vi "ActionVIOnCompile.vi"(8 "error in (no error)":errorcluster, 11 "Device Item Ref in":T1 format="%.0x") -> (0 "error out":errorcluster)   [LabVIEW 2020, in "Waveform-Processing-Custom-Device System Explorer.lvlib"]
uses:
  Waveform-Processing-Custom-Device System Explorer.lvlib
  <vilib>/NI VeriStand/Custom Device API/Custom Device Item Ref.ctl
  Shared/Types/FG Action.ctl
  Shared/CompiledSettings.ctl
  <vilib>/NI VeriStand/Custom Device API/Block Data Reference.ctl
  <vilib>/NI VeriStand/Custom Device API/Data Reference.ctl
  <vilib>/NI VeriStand/Custom Device API/Waveform Data Reference.ctl
  Shared/Constants.vi
  <vilib>/NI VeriStand/Custom Device API/Set Item Property (Variant).vi
  <vilib>/NI VeriStand/Custom Device API/Custom Device API.lvlib
  <vilib>/NI/NIVS Inline Async API/_Data Access System Explorer/Data Access System Explorer.lvlib
  Shared/Waveform-Processing-Custom-Device Shared.lvlib
  Shared/Running Average/Running Average.lvlib
  Shared/Single Point/SinglePoint.lvlib
  Shared/Scaled Waveform/Scaled Waveform.lvlib
  Shared/Debug/Debug.lvlib
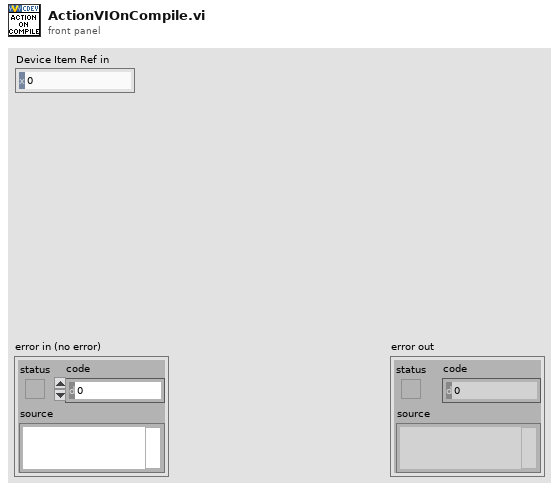
[diagram p1: front panel]
types:
  T1 = typedef "Custom Device API.lvlib/Custom Device Item Ref.ctl" = u64
  T2 = typedef "Waveform-Processing-Custom-Device Shared.lvlib/CompiledSettings.ctl" = cluster{"Name":string, "Buffer Length (samples)":u32, "Enable Array":bool[], "Parameter Block Data Refs":T3[], "Source Wfm Data Refs":T5[], "Result Wfm Data Refs":T5[], "Result Ch Data Refs":T4[], "Task Rate (Hz)":dbl}
  T3 = typedef "Custom Device API.lvlib/Block Data Reference.ctl" = cluster{"Data Reference":T4, "Offset":u64, "Length":u64}
  T4 = typedef "Custom Device API.lvlib/Data Reference.ctl" = i32
  T5 = typedef "Custom Device API.lvlib/Waveform Data Reference.ctl" = i32
  T6 = typedef "Waveform-Processing-Custom-Device Shared.lvlib/FG Action.ctl" = enum8{"GET", "SET"}
  T7 = typedef "Custom Device API.lvlib/Custom Device Item Info.ctl" = cluster{"Name":string, "Is Channel":bool, "GUID":string, "Is Waveform":bool}
  T8 = typedef "Waveform-Processing-Custom-Device Shared.lvlib/Custom Device Settings.ctl" = cluster{"CD Task Dependency":T1, "CD Task Dependency Ref":T1, "CD Task Available Wfms":string[], "CD Task Selected Wfms":string[], "Buffer Length (s)":dbl, "Buffer Length (samples)":u32, "Single-point Enabled":bool, "Running Average Enabled":bool, "Task Rate":dbl, "Scaled Waveform Enabled":bool}
  T9 = cluster{"Name":string, "Type":enum16{"Output/Write", "Input/Read", "Input/ReadWrite"}, "VS Refs":T1[]}[]
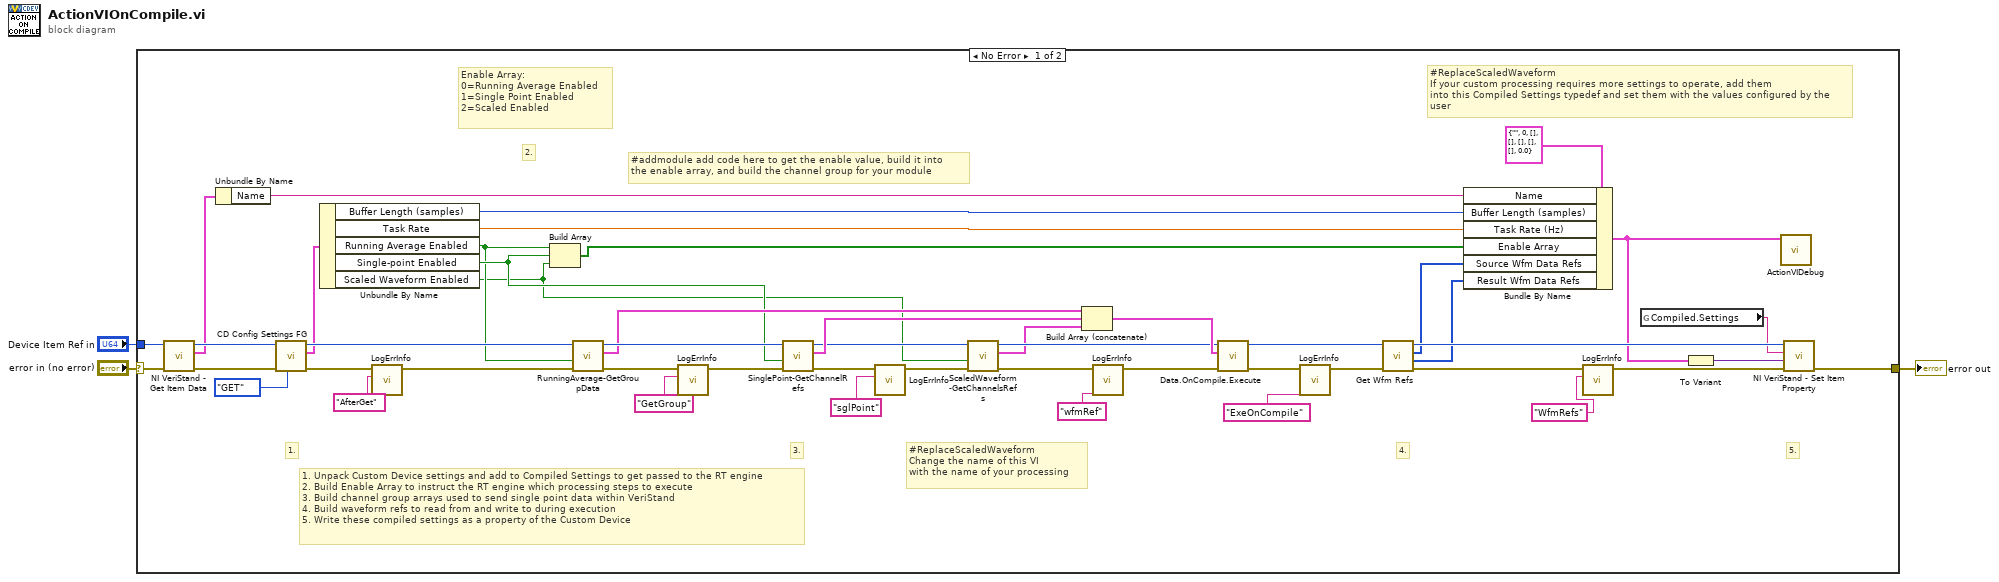
[diagram p0: block diagram]
diagram:
  n1 = case shown="No Error" "error in (no error)" {
    selector: "error in (no error)" -> [w51 w53]
    tunnel: [w52 w53] -> w2
    tunnel: "Device Item Ref in" -> [w50 _]
    frame No Error {
      # "#ReplaceScaledWaveform \nIf your custom processing requires more settings to operate, add them\ninto this Compiled Settings typedef and set them with the values configured by the user"
      # "#ReplaceScaledWaveform \nChange the name of this VI\nwith the name of your processing"
      # "#addmodule add code here to get the enable value, build it into\nthe enable array, and build the channel group for your module"
      # "Enable Array:\n0=Running Average Enabled\n1=Single Point Enabled\n2=Scaled Enabled"
      # "5."
      # "4."
      # "3."
      # "2."
      # "1."
      # "1. Unpack Custom Device settings and add to Compiled Settings to get passed to the RT engine\n2. Build Enable Array to instruct the RT engine which processing steps to execute\n3. Build channel group arrays used to send single point data within VeriStand\n4. Build waveform refs to read from and write to during execution\n5. Write these compiled settings as a property of the Custom Device"
      n2 = call <vilib>:"NI VeriStand - Get Item Data.vi"("error in (no error)"=w51, "Item Ref in"=w50) -> ("error out"=w48:errorcluster, "Item Info"=w47:T7, "Item Ref out"=w49:T1)  [unwired: 6 in, 1 out]
      n3 = Unbundle By Name(w47) -> ("Name"=w38:string)
      n4 = call "CD Config Settings FG.vi"("Action"=FG_Action."GET", "error in (no error)"=w48, "Item Ref"=w49) -> ("error out"=w16:errorcluster, "CD Settings out"=w37:T8, "Item Ref out"=w41:T1)  [unwired: 5 in, 1 out]
      n5 = Unbundle By Name(w37) -> ("Buffer Length (samples)"=w36:u32, "Task Rate"=w27:dbl, "Running Average Enabled"=w29:bool, "Single-point Enabled"=w30:bool, "Scaled Waveform Enabled"=w18:bool)
      n6 = call "LogErrInfo.vi"("location info"="AfterGet", "error in (no error)"=w16) -> ("error out"=w15:errorcluster)  [unwired: 9 in]
      n7 = Build Array(w29, w30, w18) -> (w28:bool[])
      n8 = call "RunningAverage-GetGroupData.vi"("Error in"=w15, "Enabled?"=w29, "Device Ref in"=w41) -> ("Error out"=w45:errorcluster, "Group Data Array"=w35:T9, "Device Ref out"=w40:T1)  [unwired: 6 in]
      n9 = call "LogErrInfo.vi"("location info"="GetGroup", "error in (no error)"=w45) -> ("error out"=w13:errorcluster)  [unwired: 9 in]
      n10 = call "SinglePoint-GetChannelRefs.vi"("Error in"=w13, "Enabled?"=w30, "Device Ref in"=w40) -> ("Error out"=w22:errorcluster, "Group Data Array"=w34:T9, "Device Ref out"=w19:T1)  [unwired: 6 in]
      n11 = call "LogErrInfo.vi"("location info"="sglPoint", "error in (no error)"=w22) -> ("error out"=w11:errorcluster)  [unwired: 9 in]
      n12 = call "ScaledWaveform-GetChannelsRefs.vi"("Error in"=w11, "Enabled?"=w18, "Device Ref in"=w19) -> ("Error out"=w21:errorcluster, "Group Data Array"=w17:T9, "Device Ref out"=w20:T1)  [unwired: 6 in]
      n13 = Build Array (concatenate)(w35, w34, w17) -> (w31:T9)
      n14 = call "LogErrInfo.vi"("location info"="wfmRef", "error in (no error)"=w21) -> ("error out"=w10:errorcluster)  [unwired: 9 in]
      n15 = call <vilib>:"Data.OnCompile.Execute.vi"("error in"=w10, "VS Ref Groups"=w31, "Custom Device Ref"=w20) -> ("error out"=w32:errorcluster, "Custom Device Ref"=w33:T1)  [unwired: 7 in]
      n16 = call "LogErrInfo.vi"("location info"="ExeOnCompile", "error in (no error)"=w32) -> ("error out"=w9:errorcluster)  [unwired: 9 in]
      n17 = call "Get Wfm Refs.vi"("Error in"=w9, "Device Ref in"=w33) -> ("Error out"=w44:errorcluster, "Results Wfm Data Refs"=w25:T5[], "Source Wfm Data Refs"=w26:T5[], "Device Ref out"=w39:T1)  [unwired: 6 in]
      n18 = Bundle By Name(cluster=T2 {"Name"="", "Buffer Length (samples)"=0, "Enable Array"=[], "Parameter Block Data Refs"=[], "Source Wfm Data Refs"=[], "Result Wfm Data Refs"=[], "Result Ch Data Refs"=[], "Task Rate (Hz)"=0.0} ("CompiledSettings"), "Name"=w38, "Buffer Length (samples)"=w36, "Task Rate (Hz)"=w27, "Enable Array"=w28, "Source Wfm Data Refs"=w26, "Result Wfm Data Refs"=w25) -> (w23:T2)
      n19 = call "LogErrInfo.vi"("location info"="WfmRefs", "error in (no error)"=w44) -> ("error out"=w8:errorcluster)  [unwired: 9 in]
      n20 = global read "Constants.vi" "Compiled.Settings"() -> (w24:string)
      n21 = To Variant(anything=w23) -> (Variant=w42:variant)
      n22 = call "ActionVIDebug.vi"("CompiledSettings"=w23) -> ()  [unwired: 11 in]
      n23 = call-poly <vilib>:"NI VeriStand - Set Item Property.vi"("error in (no error)"=w8, "Value"=w42, "Property Name"=w24, "Item Ref in"=w39) -> ("error out"=w52:errorcluster)  [unwired: 5 in, 2 out]
    }
    frame Error {
    }
  }
  "error out" <- w2
